vi "Execute Time Elapsed Signal.vi"(8 "error in (no error)":errorcluster, 11 "Chef Actor in":refnum<class "Chef Actor.lvclass">) -> (0 "error out":errorcluster, 3 "Chef Actor out":refnum<class "Chef Actor.lvclass">)   [LabVIEW 2024, in "Chef Actor.lvlib" / "Chef Actor.lvclass"]
uses:
  Chef Actor.lvclass
  Chef Actor.lvclass/Chef Actor.ctl
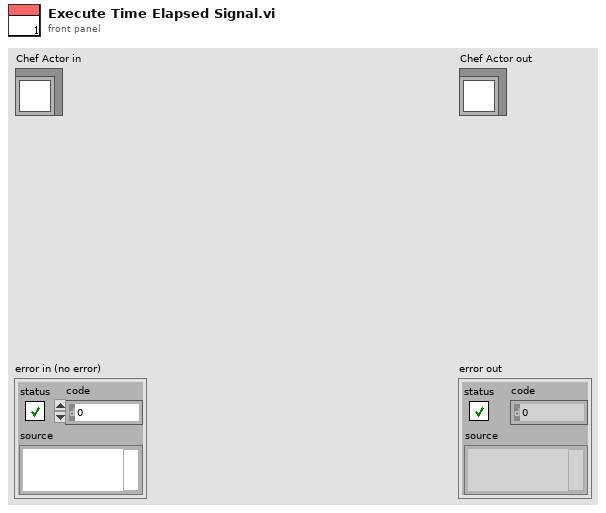
[diagram p1: front panel]
types:
  T1 = typedef "Step.ctl" = cluster{"Fire":dbl, "Duration":dbl}
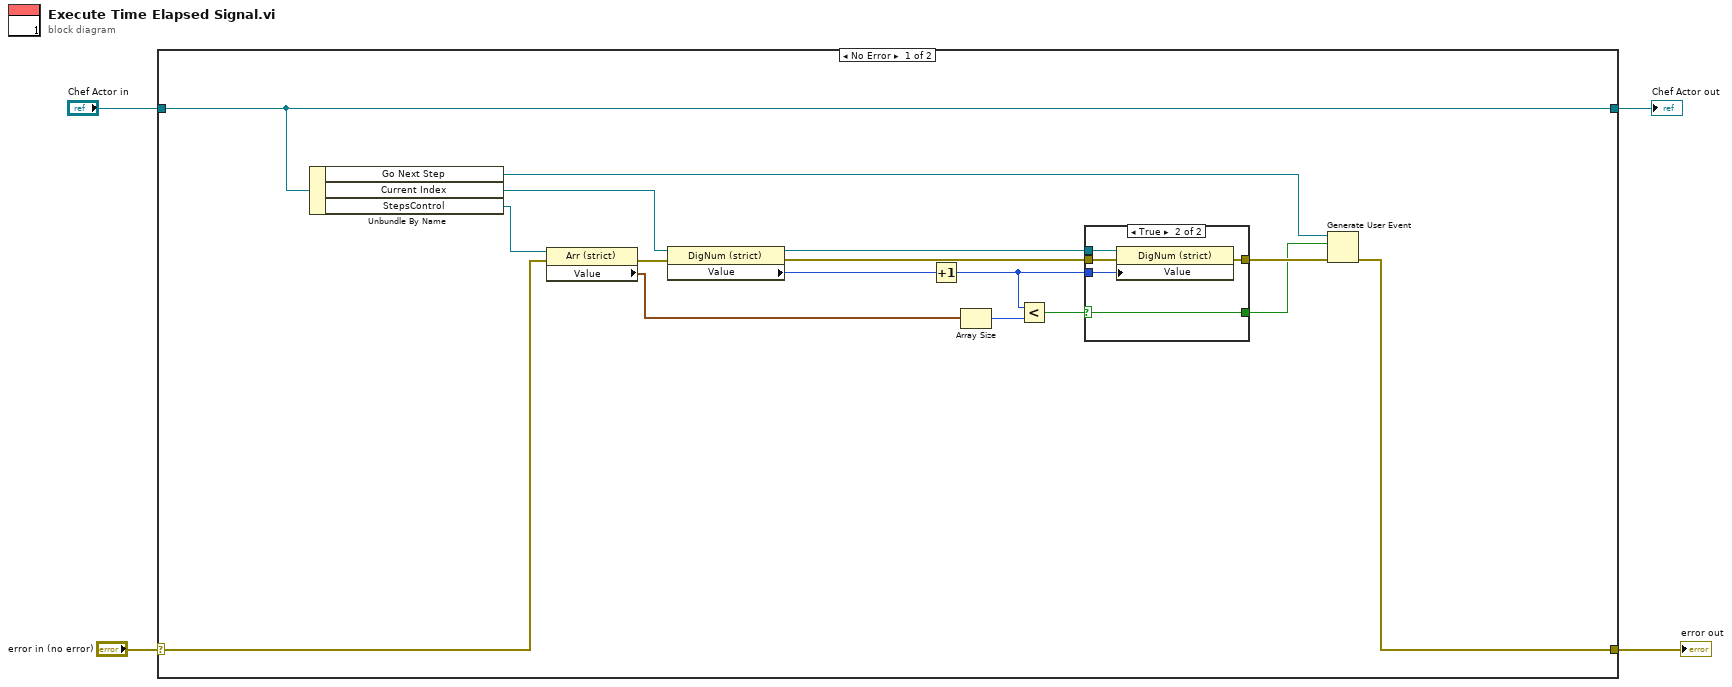
[diagram p0: block diagram]
diagram:
  n1 = case shown="No Error" "error in (no error)" {
    selector: "error in (no error)" -> [w6 w29]
    tunnel: [w5 w29] -> w3
    tunnel: [w20 w28] -> w1
    tunnel: "Chef Actor in" -> [w20 w28]
    frame No Error {
      n2 = Unbundle By Name(w20) -> ("Go Next Step"=w19:refnum<user-event>, "Current Index"=w13:refnum<vi>, "StepsControl"=w12:refnum<vi>)
      n3 = property class="Arr (strict)"(reference=w12, error in=w6) -> (error out=w16:errorcluster, "Value"=w11:T1[])  [unwired: 1 out]
      n4 = property class="DigNum (strict)"(reference=w13, error in=w16) -> (reference out=w14:refnum<vi>, error out=w15:errorcluster, "Value"=w10:i32)
      n5 = Increment(x=w10) -> (x+1=w9:i32)
      n6 = Array Size(array=w11) -> (size(s)=w18:i32)
      n7 = Less?(x=w9, y=w18) -> (x < y?=w17:bool)
      n8 = case shown="True" w17 {
        selector: w17 -> [w21 w23]
        tunnel: w15 -> [w22 w27]
        tunnel: w14 -> [_ w26]
        tunnel: w9 -> [_ w25]
        tunnel: [w22 w24] -> w8
        tunnel: [w21 w23] -> w7
        frame False {
        }
        frame True {
          n9 = property class="DigNum (strict)"(reference=w26, error in=w27, "Value"=w25) -> (error out=w24:errorcluster)  [unwired: 1 out]
        }
      }
      n10 = Generate User Event(user event=w19, event data cluster=w7, error in=w8) -> (error out=w5:errorcluster)  [unwired: 1 in, 1 out]
    }
    frame Error {
    }
  }
  "error out" <- w3
  "Chef Actor out" <- w1
